vi "Climb level 2.vi"(7 "ServoDeviceRef":T1={"DeviceStatus"={"status"=FALSE, "code"=0, "source"=""}, "PWM Channel"=enum."PWM 1", "DeadBand"={"Name"="Servo", "maxPositivePwm"=1770, "minPositivePwm"=1013, "centerPwm"=1007, "maxNegativePwm"=1000, "minNegativePwm"=243, "angularRange"=180}}, 8 "MotorControlDevRef 4":T4={"DeviceStatus"={"status"=FALSE, "code"=0, "source"=""}, "Type"=enum."PWM", "PWM"={"PWM Channel"=enum."PWM 6", "DeadBand"={"Name"="Talon", "maxPositivePwm"=1537, "minPositivePwm"=1020, "centerPwm"=1013, "maxNegativePwm"=1006, "minNegativePwm"=489, "angularRange"=0}}, "CAN"={"Device Number"=0, "SetOutput VI Ref"=variant(refnum<vi> refnum), "GetOutput VI Ref"=variant(refnum<vi> refnum), "Enable VI Ref"=variant(refnum<vi> refnum), "Disable VI Ref"=variant(refnum<vi> refnum), "Data"=variant}, "Invert"=FALSE, "DIO PWM"={"PWM \"Enable\" Channel"=enum."Invalid", "DIOChannel"=enum."Invalid", "PWM Rate"=0.0}}, 9 "MotorControlDevRef 3":T4={"DeviceStatus"={"status"=FALSE, "code"=0, "source"=""}, "Type"=enum."PWM", "PWM"={"PWM Channel"=enum."PWM 5", "DeadBand"={"Name"="Talon", "maxPositivePwm"=1537, "minPositivePwm"=1020, "centerPwm"=1013, "maxNegativePwm"=1006, "minNegativePwm"=489, "angularRange"=0}}, "CAN"={"Device Number"=0, "SetOutput VI Ref"=variant(refnum<vi> refnum), "GetOutput VI Ref"=variant(refnum<vi> refnum), "Enable VI Ref"=variant(refnum<vi> refnum), "Disable VI Ref"=variant(refnum<vi> refnum), "Data"=variant}, "Invert"=FALSE, "DIO PWM"={"PWM \"Enable\" Channel"=enum."Invalid", "DIOChannel"=enum."Invalid", "PWM Rate"=0.0}}, 10 "MotorControlDevRef 2":T4={"DeviceStatus"={"status"=FALSE, "code"=0, "source"=""}, "Type"=enum."PWM", "PWM"={"PWM Channel"=enum."PWM 4", "DeadBand"={"Name"="Talon", "maxPositivePwm"=1537, "minPositivePwm"=1020, "centerPwm"=1013, "maxNegativePwm"=1006, "minNegativePwm"=489, "angularRange"=0}}, "CAN"={"Device Number"=0, "SetOutput VI Ref"=variant(refnum<vi> refnum), "GetOutput VI Ref"=variant(refnum<vi> refnum), "Enable VI Ref"=variant(refnum<vi> refnum), "Disable VI Ref"=variant(refnum<vi> refnum), "Data"=variant}, "Invert"=FALSE, "DIO PWM"={"PWM \"Enable\" Channel"=enum."Invalid", "DIOChannel"=enum."Invalid", "PWM Rate"=0.0}}, 11 "MotorControlDevRef 1":T4={"DeviceStatus"={"status"=FALSE, "code"=0, "source"=""}, "Type"=enum."PWM", "PWM"={"PWM Channel"=enum."PWM 3", "DeadBand"={"Name"="Talon", "maxPositivePwm"=1537, "minPositivePwm"=1020, "centerPwm"=1013, "maxNegativePwm"=1006, "minNegativePwm"=489, "angularRange"=0}}, "CAN"={"Device Number"=0, "SetOutput VI Ref"=variant(refnum<vi> refnum), "GetOutput VI Ref"=variant(refnum<vi> refnum), "Enable VI Ref"=variant(refnum<vi> refnum), "Disable VI Ref"=variant(refnum<vi> refnum), "Data"=variant}, "Invert"=FALSE, "DIO PWM"={"PWM \"Enable\" Channel"=enum."Invalid", "DIOChannel"=enum."Invalid", "PWM Rate"=0.0}}) -> ()   [LabVIEW 2017]
uses:
  <vilib>/Rock Robotics/WPI/MotorControl/WPI_MotorControlDeviceRef.ctl
  <vilib>/Rock Robotics/WPI/MotorControl/WPI_MotorControlType.ctl
  <vilib>/Rock Robotics/SystemInterfaces/DIO/FPGA_DIOPWMChannel.ctl
  <vilib>/Rock Robotics/WPI/PWM/WPI_PWMDeadband.ctl
  <vilib>/Rock Robotics/SystemInterfaces/DIO/FPGA_DIOChannel.ctl
  <vilib>/Rock Robotics/WPI/PWM/Servo/WPI_ServoDeviceRef.ctl
  <vilib>/Platform/TimedLoop/XDataNode/timing_clust.ctl
  <vilib>/Platform/TimedLoop/XDataNode/nitl_modes.ctl
  <vilib>/Platform/TimedLoop/XDataNode/wakeup.ctl
  CommandTypes/Climb command.ctl
  <userlib>/836-Library/System/TDMS_V2/Support/Logging_Settings.ctl
  <userlib>/836-Library/System/TDMS_V2/Support/Group_FIFO_Config.ctl
  <userlib>/836-Library/System/TDMS_V2/Support/Channel_FIFO_Config.ctl
  <vilib>/platform/TimedLoop/XDataNode/XDataNode.xnode
  <vilib>/Platform/TimedLoop/XDataNode/XDNodeRunTimeDep.lvlib
panel:
  in  "Rev Time (s)":dbl=0.25
  in  "Reset Servo?":bool
  in  "climbSpeed":dbl=-1.0
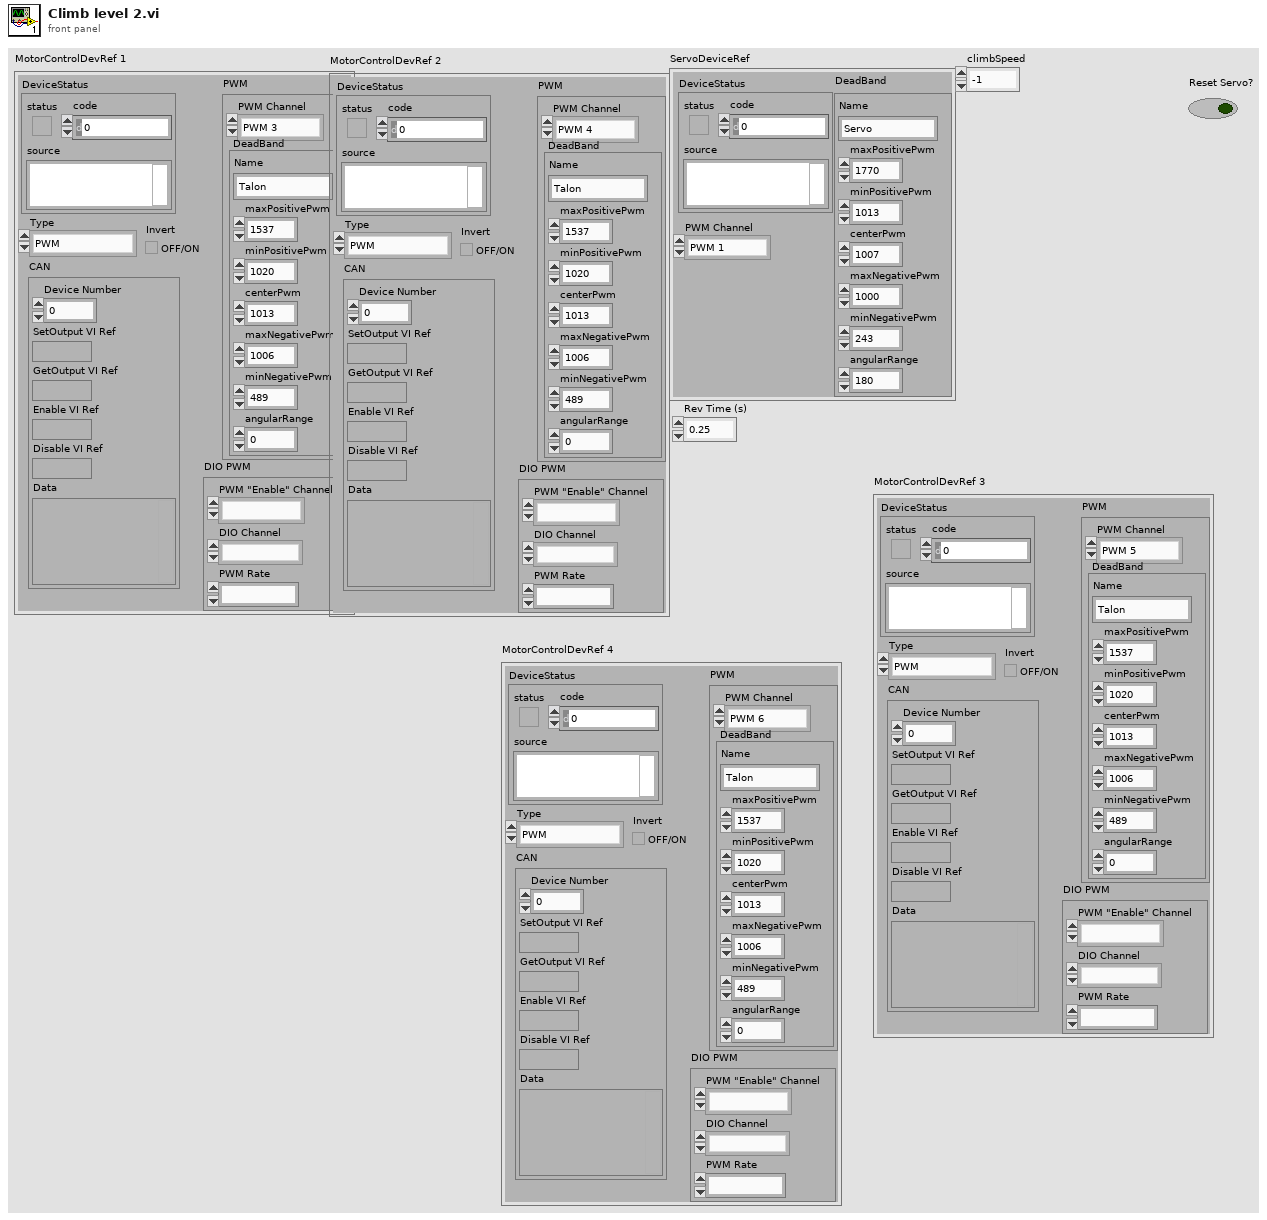
[diagram p1: front panel]
types:
  T1 = typedef "WPI_ServoDeviceRef.ctl" = cluster{"DeviceStatus":errorcluster, "PWM Channel":T2, "DeadBand":T3}
  T2 = typedef "FPGA_DIOPWMChannel.ctl" = enum8{"PWM 0", "PWM 1", "PWM 2", "PWM 3", "PWM 4", "PWM 5", "PWM 6", "PWM 7", "PWM 8", "PWM 9", "PWM MXP 0", "PWM MXP 1", "PWM MXP 2", "PWM MXP 3", "PWM MXP 4", "PWM MXP 5", "PWM MXP 6", "PWM MXP 7", "PWM MXP 8", "PWM MXP 9", "Invalid"}
  T3 = typedef "WPI_PWMDeadband.ctl" = cluster{"Name":string, "maxPositivePwm":i32, "minPositivePwm":i32, "centerPwm":i32, "maxNegativePwm":i32, "minNegativePwm":i32, "angularRange":u16}
  T4 = typedef "WPI_MotorControlDeviceRef.ctl" = cluster{"DeviceStatus":errorcluster, "Type":T5, "PWM":cluster{"PWM Channel":T2, "DeadBand":T3}, "CAN":cluster{"Device Number":u8, "SetOutput VI Ref":variant, "GetOutput VI Ref":variant, "Enable VI Ref":variant, "Disable VI Ref":variant, "Data":variant}, "Invert":bool, "DIO PWM":cluster{"PWM \"Enable\" Channel":T2, "DIOChannel":T6, "PWM Rate":dbl}}
  T5 = typedef "WPI_MotorControlType.ctl" = enum16{"PWM", "CAN", "DIO PWM"}
  T6 = typedef "FPGA_DIOChannel.ctl" = enum8{"DIO 0", "DIO 1", "DIO 2", "DIO 3", "DIO 4", "DIO 5", "DIO 6", "DIO 7", "DIO 8", "DIO 9", "DIO MXP 0", "DIO MXP 1", "DIO MXP 2", "DIO MXP 3", "DIO MXP 4", "DIO MXP 5", "DIO MXP 6", "DIO MXP 7", "DIO MXP 8", "DIO MXP 9", "DIO MXP 10", "DIO MXP 11", "DIO MXP 12", "DIO MXP 13", "DIO MXP 14", "DIO MXP 15", "SPI Port CS1", "SPI Port CS2", "SPI Port CS3", "SPI Port MISO", "SPI Port MOSI", "Invalid"}
  T7 = typedef "XDNodeRunTimeDep.lvlib/timing_clust.ctl" = cluster{"Expected End [f-1]":u64, "Actual End [f-1]":u64, "Finished Late? [f-1]":bool, "Expected End [i-1]":u64, "Actual End [i-1]":u64, "Finished Late? [i-1]":bool, "Expected Start [i]":u64, "Actual Start [i]":u64, "Expected Start [f]":u64, "Actual Start [f]":u64, "Source Name":string, "Structure Name":string, "Period":i64, "Deadline":i64, "Offset":i64, "Start":i64, "Priority":i32, "Timeout":i32, "Mode":T8, "Wakeup Reason":T9, "Error":errorcluster, "Source Type":string, "Secondary Source Type":string, "Global End Time":u64, "Global Start Time":u64, "Frame Duration":u64, "Iteration Duration":u64, "Assigned CPU":i32, "I/O Scan Engine Mode":u32}
  T8 = typedef "XDNodeRunTimeDep.lvlib/nitl_modes.ctl" = enum32{"No Change", "Process missed periods, maintain original phase", "Discard missed periods, maintain original phase", "Process missed periods, ignore original phase", "Discard missed periods, ignore original phase"}
  T9 = typedef "XDNodeRunTimeDep.lvlib/wakeup.ctl" = enum32{"Normal", "Aborted", "Asynchronous wakeup", "Timing source error", "Timed loop error", "Timeout"}
  T10 = typedef "Climb command.ctl" = enum16{"Do Nothing", "Deploy", "Winch"}
  T11 = typedef "Logging_Settings.ctl" = cluster{"Data Grab Period":dbl, "File Write Period":dbl, "Max Stored Size":dbl, "Burst Size":dbl}
  T12 = typedef "Group_FIFO_Config.ctl" = cluster{"Group":string, "Channels":T13[], "Channel Names":string[]}
  T13 = typedef "Channel_FIFO_Config.ctl" = cluster{"Channel":string, "FIFO":refnum<k33>}
  T14 = typedef "Semaphore RefNum" = refnum<k1>
  T15 = cluster{"Name":string, "File Ref":refnum<k34>, "Start Time":timestamp, "Logging Settings":T11, "Group FIFO Config":T12[], "Data To Write":refnum<data-value>, "semaphore":T14}
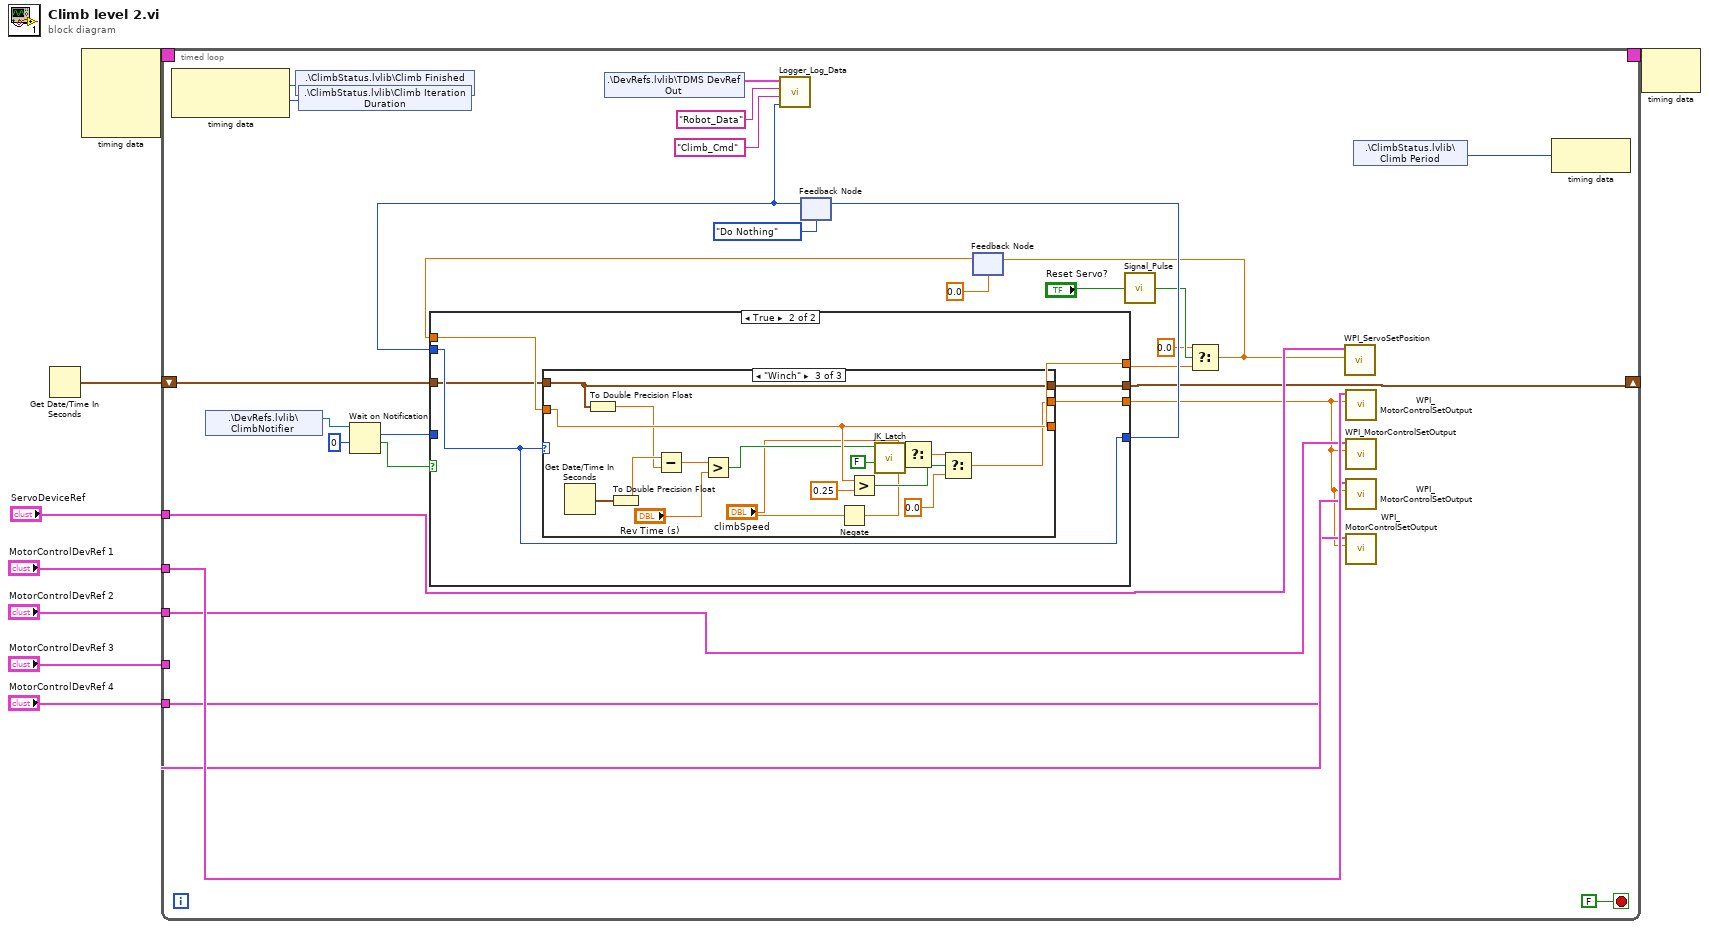
[diagram p0: block diagram]
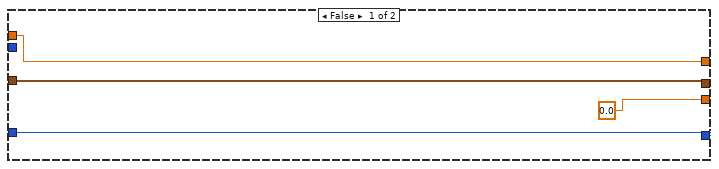
[diagram p2: hidden frame]
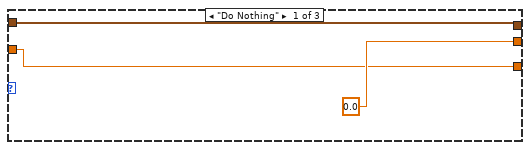
[diagram p3: hidden frame]
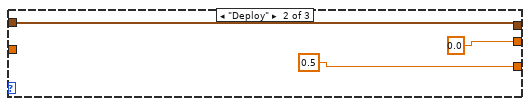
[diagram p4: hidden frame]
diagram:
  n1 = Get Date/Time In Seconds() -> (seconds since 1Jan1904=w1:timestamp)
  n2 = node-c288() -> (w8:T7)  [unwired: 4 in]
  n3 = timed-loop {
    timing: w8 -> [_]
    timing-out: [_] -> w7
    tunnel: "MotorControlDevRef 1" -> [w33]
    tunnel: "MotorControlDevRef 2" -> [w32]
    tunnel: "MotorControlDevRef 3" -> [w31]
    tunnel: "MotorControlDevRef 4" -> [w30]
    tunnel: "ServoDeviceRef" -> [w28]
    shift-right: [w13] -> _
    shift-left: w1 -> [w14]
    stop <- FALSE stop-if-true
    n4 = node-c288() -> (w21:bool, w20:i64)  [unwired: 1 in]
    n5 = shared-variable ".\\DevRefs.lvlib\\ClimbNotifier"() -> (w23:refnum<notifier>)  [unwired: 1 in, 1 out]
    n6 = shared-variable ".\\ClimbStatus.lvlib\\Climb Finished Late? [i-1]"(w21) -> ()  [unwired: 1 in, 1 out]
    n7 = shared-variable ".\\ClimbStatus.lvlib\\Climb Iteration Duration"(w20) -> ()  [unwired: 1 in, 1 out]
    n8 = Wait on Notification(notifier=w23, timeout in ms (-1)=0) -> (notification=w35:enum16{"Do Nothing", "Deploy", "Winch"}, timed out?=w36:bool)  [unwired: 2 in, 2 out]
    n9 = shared-variable ".\\DevRefs.lvlib\\TDMS DevRef Out"() -> (w12:T15)  [unwired: 1 in, 1 out]
    n10 = feedback #1(Climb_command."Do Nothing") -> (w9:T10)
    n11 = call <userlib>:"Logger_Log_Data.vi"("Data"=w9, "Channel"="Climb_Cmd", "Group"="Robot_Data", "TDMS DevRef"=w12) -> ()  [unwired: 7 in, 1 out]
    n12 = feedback #2(0.0) -> (w25:dbl)
    n13 = case shown="True" w36 {
      tunnel: w35 -> [w41 _]
      tunnel: [w41 w44] -> w34
      tunnel: w9 -> [_ w44]
      tunnel: [0.0 w47] -> w27
      tunnel: w25 -> [w39 w46]
      tunnel: [w39 w45] -> w17
      tunnel: w14 -> [w38 w43]
      tunnel: [w38 w42] -> w13
      frame False {
      }
      frame True {
        n14 = case shown="\"Winch\"" w44 {
          tunnel: [0.0 0.0 w67] -> w47
          tunnel: w46 -> [w49 _ w69]
          tunnel: [w49 0.5 w69] -> w45
          tunnel: w43 -> [w48 w51 w63]
          tunnel: [w48 w51 w63] -> w42
          frame "Do Nothing" {
          }
          frame "Deploy" {
          }
          frame "Winch" {
            n15 = Get Date/Time In Seconds() -> (seconds since 1Jan1904=w62:timestamp)
            n16 = To Double Precision Float(number=w63) -> (double precision float=w60:dbl)
            n17 = To Double Precision Float(number=w62) -> (double precision float=w61:dbl)
            n18 = Subtract(x=w61, y=w60) -> (x-y=w59:dbl)
            n19 = Greater?(x=w59, y="Rev Time (s)") -> (0:w57:bool)
            n20 = Negate(x="climbSpeed") -> (-x=w54:dbl)
            n21 = Greater?(x=w69, y=0.25) -> (0:w68:bool)
            n22 = call <userlib>:"JK_Latch.vi"("Reset"=FALSE, "Set"=w57) -> ("Q"=w64:bool)  [unwired: 5 in]
            n23 = Select(t="climbSpeed", s=w64, f=w54) -> (s? t:f=w65:dbl)
            n24 = Select(t=w65, s=w68, f=0.0) -> (s? t:f=w67:dbl)
          }
        }
      }
    }
    n25 = feedback-in #1(w34) -> ()
    n26 = call <userlib>:"Signal_Pulse.vi"("Input"="Reset Servo?") -> ("Output"=w16:bool)
    n27 = Select(t=0.0, s=w16, f=w17) -> (s? t:f=w18:dbl)
    n28 = feedback-in #2(w18) -> ()
    n29 = call <vilib>:"WPI_ServoSetPosition.vi"("Position"=w18, "ServoDeviceRef"=w28) -> ()  [unwired: 8 in, 2 out]
    n30 = call <vilib>:"WPI_MotorControlSetOutput.vi"("Output"=w27, "MotorControlDevRef"=w33) -> ()  [unwired: 7 in, 3 out]
    n31 = call <vilib>:"WPI_MotorControlSetOutput.vi"("Output"=w27, "MotorControlDevRef"=w32) -> ()  [unwired: 7 in, 3 out]
    n32 = call <vilib>:"WPI_MotorControlSetOutput.vi"("Output"=w27, "MotorControlDevRef"=w31) -> ()  [unwired: 7 in, 3 out]
    n33 = call <vilib>:"WPI_MotorControlSetOutput.vi"("Output"=w27, "MotorControlDevRef"=w30) -> ()  [unwired: 7 in, 3 out]
    n34 = shared-variable ".\\ClimbStatus.lvlib\\Climb Period"() -> (w22:i64)  [unwired: 1 in, 1 out]
    n35 = node-c288(w22) -> ()  [unwired: 1 out]
  }
  n36 = node-c288(w7) -> ()  [unwired: 1 out]
